vi "UDP.vi"(5 "In":u8=255 format="%.0x", 6 "timeout ms (2000)":i32=2000, 7 "error in (no error)":errorcluster, 8 "Read (TRUE)":bool, 9 "Address":u32=64 format="%.0x", 10 "IP address":string="192.168.10.20") -> (0 "error out":errorcluster={"status"=TRUE, "code"=56, "source"="UDP Read in UDP.vi->flash.vi"}, 1 "Out":u8 format="%.0x", 2 "received string":string)   [LabVIEW 2017]
panel:
  out "字符串":string
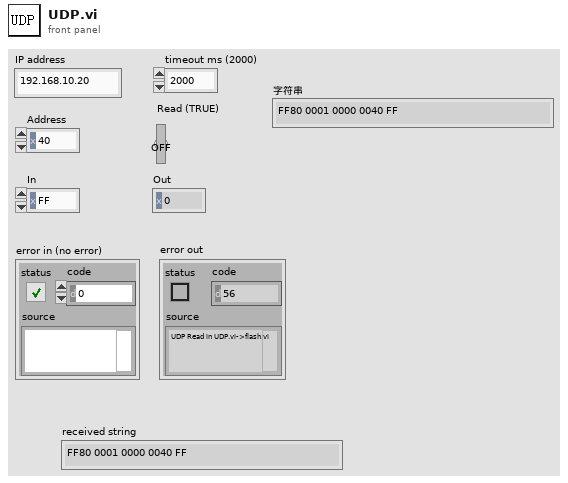
[diagram p1: front panel]
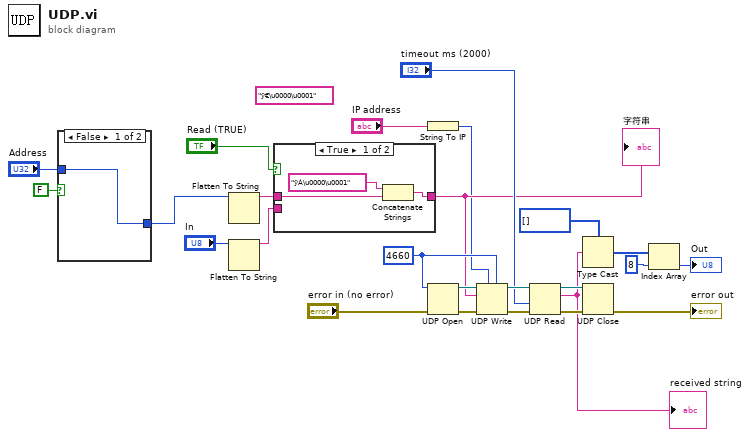
[diagram p0: block diagram]
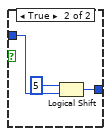
[diagram p2: hidden frame]
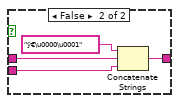
[diagram p3: hidden frame]
diagram:
  (unwired) "ÿ€\u0000\u0001" ("initial string")
  w22 = u16 4660 ("UDP port")
  n1 = case shown="False" FALSE {
    tunnel: [w26 w28] -> w4
    tunnel: "Address" -> [w26 w27]
    frame False {
    }
    frame True {
      n2 = Logical Shift(y=i16 5, x=w27) -> (x << y=w28:u32)
    }
  }
  n3 = Flatten To String(anything=w4) -> (data string=w15:string)  [unwired: 3 in, 2 out]
  n4 = Flatten To String(anything="In") -> (data string=w13:string)  [unwired: 3 in, 2 out]
  n5 = case shown="True" "Read (TRUE)" {
    tunnel: [w31 w35] -> w16
    tunnel: w15 -> [w30 w34]
    tunnel: w13 -> [_ w33]
    frame True {
      n6 = Concatenate Strings("ÿÀ\u0000\u0001" ("initial string"), w30) -> (w31:string)
    }
    frame False {
      n7 = Concatenate Strings("ÿ€\u0000\u0001" ("initial string"), w34, w33) -> (w35:string)
    }
  }
  "字符串" <- w16
  n8 = String To IP(1:"IP address") -> (0:w6:u32)
  n9 = UDP Open(8:"error in (no error)", 11:w22) -> (port=w24:refnum<k16>, 0:w23:errorcluster)  [unwired: 3 in, 1 out]
  n10 = UDP Write(address=w6, port or service name=w22, connection ID=w24, data in=w16, 8:w23) -> (error out=w19:errorcluster, 3:w21:refnum<k16>)  [unwired: 1 in]
  n11 = UDP Read(connection ID=w21, timeout ms (25000)="timeout ms (2000)", 8:w19) -> (data out=w1:string, error out=w18:errorcluster, 3:w20:refnum<k16>)  [unwired: 3 out]
  "received string" <- w1
  n12 = Type Cast(type=u8[] [], x=w1) -> (*(type *) &x=w10:u8[])
  n13 = UDP Close(connection ID=w20, 8:w18) -> (error out=→"error out":errorcluster)  [unwired: 1 out]
  n14 = Index Array(array=w10, index=8) -> (element=→"Out":u8)
